vi "player.vi"() -> ()   [LabVIEW 2017]
uses:
  <vilib>/express/express analysis/Spectral/Block/exnSpectralBlock spectral measurements peak poly.vi
  <vilib>/express/express analysis/Spectral/Block/exnSpectralBlock spectral measurements peak DDT.vi
  <vilib>/sound2/lvsound2.llb/Sound File Write Open.vi
  <vilib>/sound2/lvsound2.llb/Sound File Write (DBL).vi
  <vilib>/express/express analysis/Spectral/XNode/ExpressSpectralMeasurementsBlockNode.xnode
panel:
  in  "关闭按钮":boolean
  in  "菜单":T1
  in  "转盘":knob scale=4000.0..10000.0 scale format="%#_5g"
  out "波形图表 3":graph
  out "文件名：":string
  in  "右声道音量":slide scale=0.0..100.0
  out "幅\n度\nV":graph caption="频谱图"
  in  "刷新按钮":boolean
  in  "左声道音量":slide scale=0.0..100.0
  in  "Player":container caption="WindowsMediaPlayer"
  in  "通道":boolean caption="通道关闭按钮"
  in  "文件路径":path caption="文件路径："
  out "波形图表 4":graph
  out "波形图表 2":graph
  out "记录状态:":boolean
  out "记录时间：":numeric format="%<%H:%M:%S>t"
  out "波形图表":graph
  in  "声道选择：":ring items=["左", "右", "双"]
  in  "采样精度：":ring items=["16", "8"]
  in  "文件名称：":string
  in  "停止按钮":boolean
  in  "录音按钮":boolean
  in  "文件夹名：":path
  in  "采样频率：":ring items=["22050", "44100"]
  # "通用音乐播放器"
  # "由测控1503班邓益宇（0904150304）制作"
  # "请点击选择功能："
  # "请在切换功能时注意myDAQ的AUDIO IN 连接线！"
  # "左\n声\n道\n声\n强"
  # "右\n声\n道声强"
  # "高\n频\n上\n限\nHz"
  # "录音配置："
  # "左\n声\n道\n波\n形"
  # "声道"
  # "Hz"
  # "位"
  # ".wav"
  # "右\n声\n道\n波\n形"
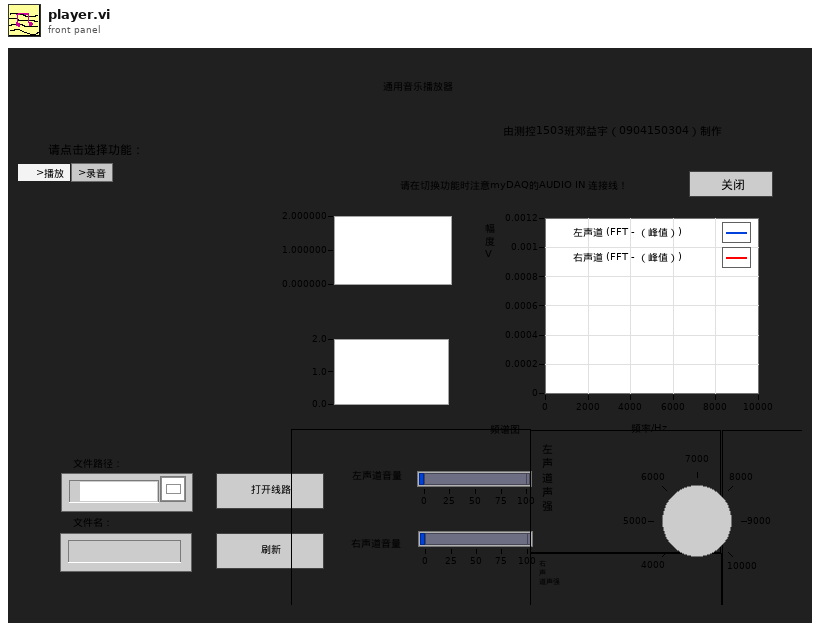
[diagram p1: front panel]
types:
  T1 = tab{"?":ring items=["    >播放", ">录音"], "转盘":knob, "波形图表 3":graph, "文件名：":string, "右声道音量":slide, "幅\n度\nV":graph, "刷新按钮":boolean, "左声道音量":slide, "Player":container, "通道":boolean, "文件路径":path, "波形图表 4":graph, "波形图表 2":graph, "记录状态:":boolean, "记录时间：":numeric, "波形图表":graph, "声道选择：":ring items=["左", "右", "双"], "采样精度：":ring items=["16", "8"], "文件名称：":string, "停止按钮":boolean, "录音按钮":boolean, "文件夹名：":path, "采样频率：":ring items=["22050", "44100"]}
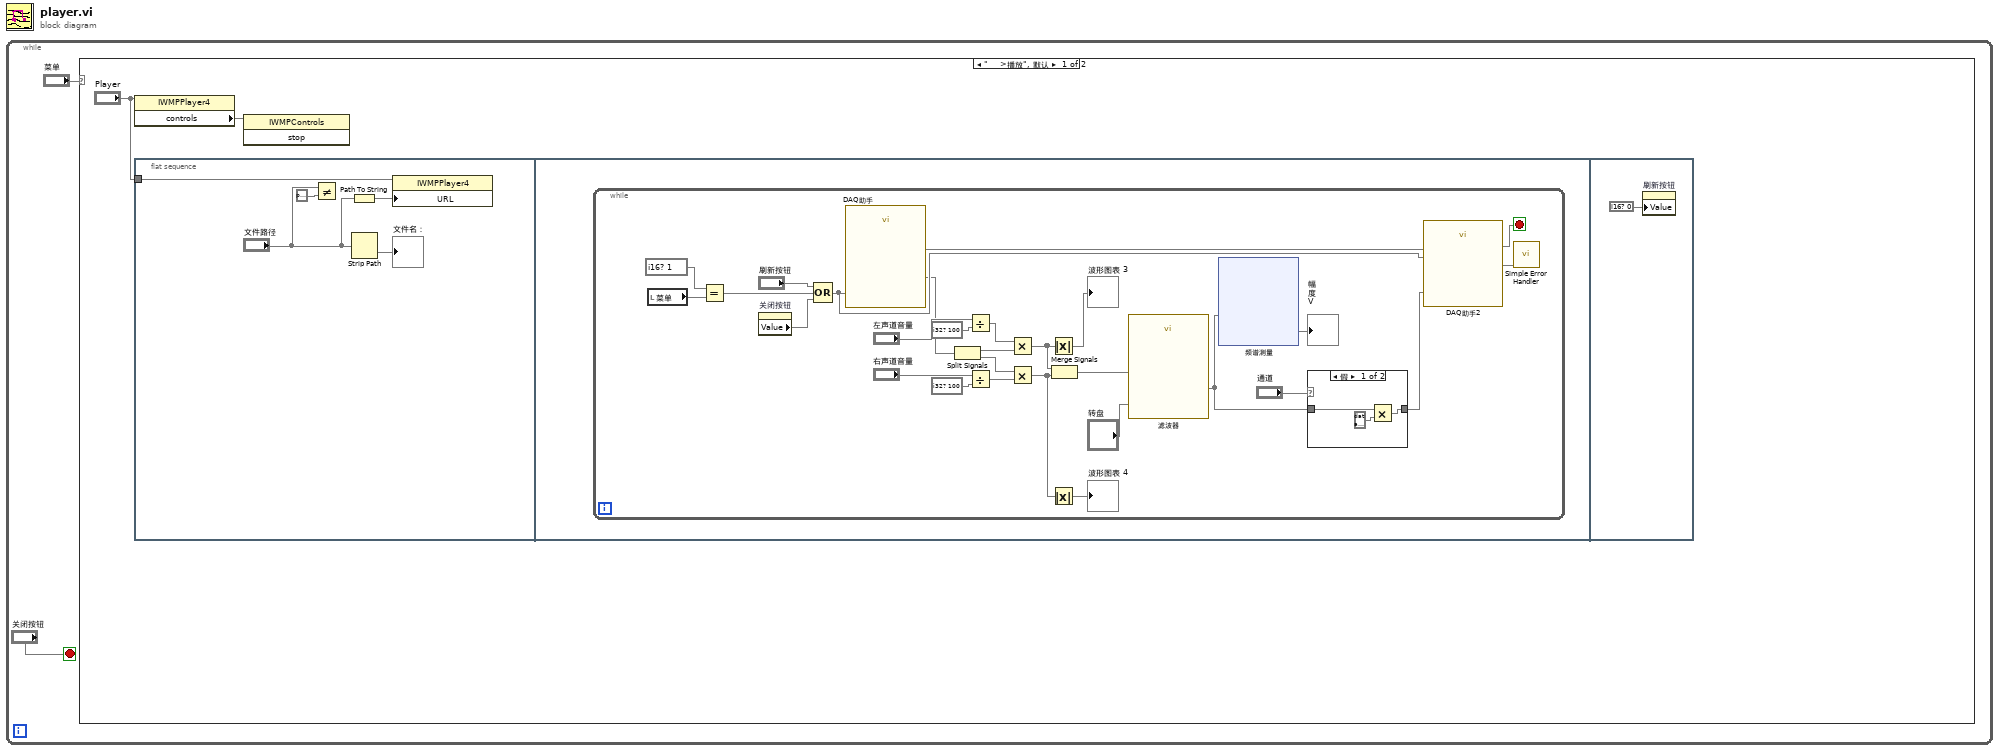
[diagram p0: block diagram]
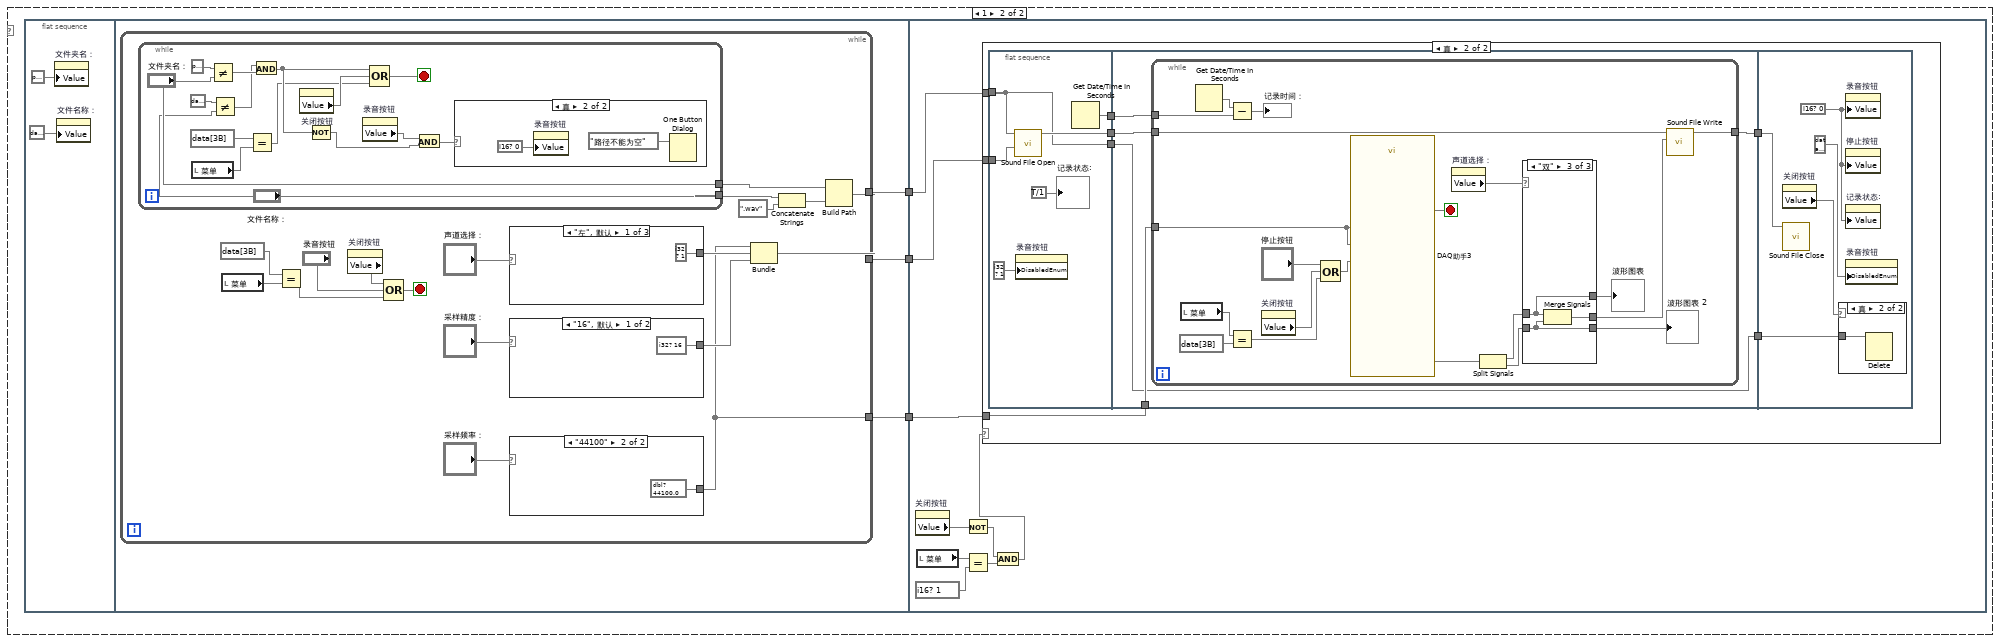
[diagram p3: hidden frame]
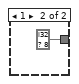
[diagram p5: hidden frame]
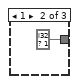
[diagram p6: hidden frame]
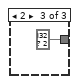
[diagram p7: hidden frame]
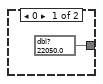
[diagram p8: hidden frame]
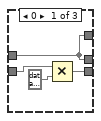
[diagram p10: hidden frame]
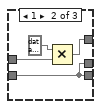
[diagram p11: hidden frame]
diagram:
  n1 = while {
    stop <- "关闭按钮" stop-if-true
    n2 = case shown="\"    >播放\", 默认" "菜单" {
      frame 0 {
        n3 = property class="IWMPPlayer4"(reference="Player") -> ("controls"=w4)  [unwired: 1 in, 2 out]
        n4 = flat-sequence {
          tunnel: "Player" -> [w9]
          frame #0 {
            n5 = Not Equal?(x="文件路径", y=path "") -> ()  [unwired: 1 out]
            n6 = Path To String(path="文件路径") -> (string=w8)
            n7 = Strip Path(path="文件路径") -> (name=→"文件名：")  [unwired: 1 out]
            n8 = property on="属性节点" class="IWMPPlayer4"(reference=w9, "URL"=w8) -> ()  [unwired: 1 in, 2 out]
          }
          frame #1 {
            n9 = while {
              stop <- w23 stop-if-true
              w37 = i16? 1 items=["播放", "录音"]
              n10 = local read "菜单"() -> (w18)
              n11 = Equal?(x=w37, y=w18) -> (x = y?=w36)
              n12 = property on="关闭按钮" class="Bool (严格)"() -> ("Value"=w20)  [unwired: 2 in, 2 out]
              n13 = Compound Arithmetic op=OR ("复合运算")("刷新按钮", w36, w20) -> (w32)
              n14 = call "DAQ助手"(7:w32) -> (15:w25, 19:w11)  [unwired: 15 in, 2 out]
              n15 = Split Signals(w25) -> (w27, w28)  [unwired: 2 in]
              n16 = Divide(x="左声道音量", y=i32? 100) -> (x/y=w31)
              n17 = Divide(x="右声道音量", y=i32? 100) -> (x/y=w34)
              n18 = Multiply(x=w31, y=w27) -> (x*y=w15)
              n19 = Multiply(x=w28, y=w34) -> (x*y=w12)
              n20 = Absolute Value(x=w15) -> (abs(x)=→"波形图表 3")
              n21 = Absolute Value(x=w12) -> (abs(x)=→"波形图表 4")
              n22 = Merge Signals(w15, w12) -> (w17)
              n23 = call "滤波器"(9:"转盘", 11:w17) -> (3:w16)  [unwired: 8 in, 1 out]
              n24 = xnode "频谱测量"(w16) -> (→"幅\n度\nV")  [unwired: 1 in, 2 out]
              n25 = case shown="假" "通道" {
                tunnel: w16 -> [w40 w41]
                tunnel: [w39 w41] -> w21
                frame 0 {
                  n26 = Multiply(x=w40, y=data[5B]) -> (x*y=w39)
                }
                frame 1 {
                }
              }
              n27 = call "DAQ助手2"(1:w21, 5:w11, 7:w32) -> (18:w23, 19:w19)  [unwired: 14 in, 1 out]
              n28 = call <vilib>:"Simple Error Handler.vi"(9:w19) -> ()  [unwired: 4 in, 5 out]
            }
          }
          frame #2 {
            n29 = property on="刷新按钮" class="Bool (严格)"("Value"=i16? 0) -> ()  [unwired: 2 in, 2 out]
          }
        }
        n30 = invoke class="IWMPControls" method="stop"(reference=w4) -> ()  [unwired: 2 in, 3 out]
      }
      frame 1 {
        n31 = flat-sequence {
          tunnel: [w60] -> w55
          tunnel: [w59] -> w54
          tunnel: [w58] -> w53
          tunnel: w55 -> [w111]
          tunnel: w54 -> [w109]
          tunnel: w53 -> [w110]
          frame #0 {
            n32 = property on="文件夹名：" class="Path"("Value"=path "") -> ()  [unwired: 2 in, 2 out]
            n33 = property on="文件名称：" class="Str"("Value"=data[5B]) -> ()  [unwired: 2 in, 2 out]
          }
          frame #1 {
            n34 = while {
              tunnel: [w68] -> w60
              tunnel: [w69] -> w59
              tunnel: [w67] -> w58
              stop <- w66 stop-if-true
              w63 = data[3B] items=["播放", "录音"]
              n35 = while {
                tunnel: ["文件夹名："] -> w73
                tunnel: ["文件名称："] -> w70
                stop <- w82 stop-if-true
                w81 = data[3B] items=["播放", "录音"]
                n36 = local read "菜单"() -> (w80)
                n37 = Not Equal?(x=path "", y="文件夹名：") -> (x != y?=w90)
                n38 = Not Equal?(x=data[5B], y="文件名称：") -> (x != y?=w89)
                n39 = Equal?(x=w81, y=w80) -> (x = y?=w79)
                n40 = And ("与")(x=w89, y=w90) -> (x .and. y?=w84)
                n41 = property on="关闭按钮" class="Bool (严格)"() -> ("Value"=w83)  [unwired: 2 in, 2 out]
                n42 = Not(x=w84) -> (.not. x?=w86)
                n43 = property on="录音按钮" class="Bool (严格)"() -> ("Value"=w87)  [unwired: 2 in, 2 out]
                n44 = Compound Arithmetic op=OR(w84, w83, w79) -> (w82)
                n45 = And(x=w87, y=w86) -> (x .and. y?=w85)
                n46 = case shown="真" w85 {
                  frame 0 {
                  }
                  frame 1 {
                    n47 = property on="录音按钮" class="Bool (严格)"("Value"=i16? 0) -> ()  [unwired: 2 in, 2 out]
                    n48 = One Button Dialog(message="路径不能为空") -> ()  [unwired: 1 in, 1 out]
                  }
                }
              }
              n49 = local read "菜单"() -> (w62)
              n50 = Equal?(x=w63, y=w62) -> (x = y?=w61)
              n51 = property on="关闭按钮" class="Bool (严格)"() -> ("Value"=w65)  [unwired: 2 in, 2 out]
              n52 = Compound Arithmetic op=OR(w65, "录音按钮", w61) -> (w66)
              n53 = case shown="\"左\", 默认" "声道选择：" {
                tunnel: [i32? 1 i32? 1 i32? 2] -> w76
                frame 0 {
                }
                frame 1 {
                }
                frame 2 {
                }
              }
              n54 = case shown="\"16\", 默认" "采样精度：" {
                tunnel: [i32? 16 i32? 8] -> w74
                frame 0 {
                }
                frame 1 {
                }
              }
              n55 = case shown="\"44100\"" "采样频率：" {
                tunnel: [dbl? 22050.0 dbl? 44100.0] -> w69
                frame 0 {
                }
                frame 1 {
                }
              }
              n56 = Bundle(w69, w76, w74) -> (w67)  [unwired: 1 in]
              n57 = Concatenate Strings(w70, ".wav") -> (w71)
              n58 = Build Path(base path=w73, name or relative path=w71) -> (appended path=w68)
            }
          }
          frame #2 {
            w108 = i16? 1 items=["播放", "录音"]
            n59 = property on="关闭按钮" class="Bool (严格)"() -> ("Value"=w105)  [unwired: 2 in, 2 out]
            n60 = local read "菜单"() -> (w107)
            n61 = Not(x=w105) -> (.not. x?=w104)
            n62 = Equal?(x=w107, y=w108) -> (x = y?=w106)
            n63 = And(x=w104, y=w106) -> (x .and. y?=w103)
            n64 = case shown="真" w103 {
              tunnel: w111 -> [_ w119]
              tunnel: w110 -> [_ w118]
              tunnel: w109 -> [_ w116]
              frame 0 {
              }
              frame 1 {
                n65 = flat-sequence {
                  tunnel: w119 -> [w122]
                  tunnel: w118 -> [w125]
                  tunnel: [w124] -> w117
                  tunnel: [w123] -> w114
                  tunnel: [w122] -> w112
                  tunnel: w117 -> [w130]
                  tunnel: w116 -> [w129]
                  tunnel: [w128] -> w115
                  tunnel: w114 -> [w127]
                  tunnel: [w126] -> w113
                  tunnel: w112 -> [w126]
                  tunnel: w115 -> [w165]
                  tunnel: w113 -> [w164]
                  frame #0 {
                    n66 = call-poly <vilib>:"Sound File Open.vi"(9:w125, 11:w122) -> (3:w124)  [unwired: 8 in, 1 out]
                    n67 = property on="录音按钮" class="Bool (严格)"("DisabledEnum"=i32? 1) -> ()  [unwired: 2 in, 2 out]
                    n68 = Get Date/Time In Seconds() -> (seconds since 1Jan1904=w123)
                    "记录状态:" <- T/1
                  }
                  frame #1 {
                    n69 = while {
                      tunnel: [w149] -> w128
                      tunnel: w130 -> [w142]
                      tunnel: w129 -> [w141]
                      tunnel: w127 -> [w134]
                      stop <- w150 stop-if-true
                      w140 = data[3B] items=["播放", "录音"]
                      n70 = local read "菜单"() -> (w139)
                      n71 = Get Date/Time In Seconds() -> (seconds since 1Jan1904=w135)
                      n72 = Subtract(x=w135, y=w134) -> (x-y=→"记录时间：")
                      n73 = Equal?(x=w139, y=w140) -> (x = y?=w138)
                      n74 = property on="关闭按钮" class="Bool (严格)"() -> ("Value"=w143)  [unwired: 2 in, 2 out]
                      n75 = Compound Arithmetic op=OR("停止按钮", w143, w138) -> (w145)
                      n76 = call "DAQ助手3"(2:w141, 3:w141, 7:w145) -> (15:w137, 18:w150)  [unwired: 13 in, 2 out]
                      n77 = property on="声道选择：" class="Enum (严格)"() -> ("Value"=w148)  [unwired: 2 in, 2 out]
                      n78 = Split Signals(w137) -> (w147, w146)  [unwired: 2 in]
                      n79 = case shown="\"双\"" w148 {
                        tunnel: [w154 w155 w159] -> w132
                        tunnel: w147 -> [w151 w158 w160]
                        tunnel: w146 -> [w153 w155 w159]
                        tunnel: [w151 w157 w160] -> w133
                        tunnel: [w151 w155 w161] -> w131
                        frame 0 {
                          n80 = Multiply(x=w153, y=data[5B]) -> (x*y=w154)
                        }
                        frame 1 {
                          n81 = Multiply(x=data[5B], y=w158) -> (x*y=w157)
                        }
                        frame 2 {
                          n82 = Merge Signals(w160, w159) -> (w161)
                        }
                      }
                      "波形图表" <- w133
                      "波形图表 2" <- w132
                      n83 = call-poly <vilib>:"Sound File Write.vi"(10:w131, 11:w142) -> (3:w149)  [unwired: 8 in, 1 out]
                    }
                  }
                  frame #2 {
                    w163 = i16? 0
                    n84 = property on="关闭按钮" class="Bool (严格)"() -> ("Value"=w166)  [unwired: 2 in, 2 out]
                    n85 = call <vilib>:"Sound File Close.vi"(11:w165) -> ()  [unwired: 10 in, 1 out]
                    n86 = case shown="真" w166 {
                      tunnel: w164 -> [_ w167]
                      frame 0 {
                      }
                      frame 1 {
                        n87 = Delete(path (use dialog)=w167) -> ()  [unwired: 4 in, 3 out]
                      }
                    }
                    n88 = property on="录音按钮" class="Bool (严格)"("Value"=w163) -> ()  [unwired: 2 in, 2 out]
                    n89 = property on="停止按钮" class="Bool (严格)"("Value"=w163) -> ()  [unwired: 2 in, 2 out]
                    n90 = property on="记录状态:" class="Bool (严格)"("Value"=w163) -> ()  [unwired: 2 in, 2 out]
                    n91 = property on="录音按钮" class="Bool (严格)"("DisabledEnum"=data[5B]) -> ()  [unwired: 2 in, 2 out]
                  }
                }
              }
            }
          }
        }
      }
    }
  }
